vi "Register Process.vi"(0 "Message Handler In":refnum<class "Message Handler.lvclass">, 1 "ProcessRefs":T1, 7 "Process":refnum<class "ICanCommunicate.lvclass">, 11 "Error In":errorcluster) -> (4 "Message Handler Out":refnum<class "Message Handler.lvclass">, 15 "Error Out":errorcluster)   [LabVIEW 2023, in "Message Handler.lvclass"]
uses:
  Message Handler.lvclass
  Interfaces/ICanCommunicate/ICanCommunicate.lvclass
  Interfaces/ICanCommunicate/Process Refs.ctl
  Interfaces/ICanCommunicate/ToProcessQueue.ctl
  Interfaces/ICanCommunicate/Message.ctl
  Interfaces/ICanCommunicate/FromProcessQueue.ctl
  Interfaces/ICanCommunicate/ProcessSyncQueue.ctl
  Private/Ctrls/Registration Data.ctl
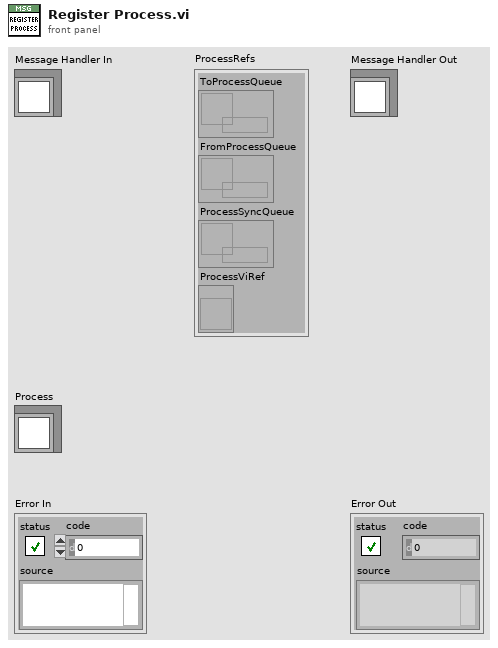
[diagram p1: front panel]
types:
  T1 = typedef "ICanCommunicate.lvclass/Process Refs.ctl" = cluster{"ToProcessQueue":T2, "FromProcessQueue":T3, "ProcessSyncQueue":T4, "ProcessViRef":refnum<vi>}
  T2 = typedef "ICanCommunicate.lvclass/ToProcessQueue.ctl" = refnum<queue>
  T3 = typedef "ICanCommunicate.lvclass/FromProcessQueue.ctl" = refnum<queue>
  T4 = typedef "ICanCommunicate.lvclass/ProcessSyncQueue.ctl" = refnum<queue>
  T5 = typedef "Message Handler.lvclass/Registration Data.ctl" = cluster{"ICanCommunicate":refnum<class "ICanCommunicate.lvclass">, "ProcessRefs":T1}
  T6 = typedef "ICanCommunicate.lvclass/Message.ctl" = cluster{"Sender Name":string, "Recipent Name":string, "Command":string, "Data":variant, "Signature":string}
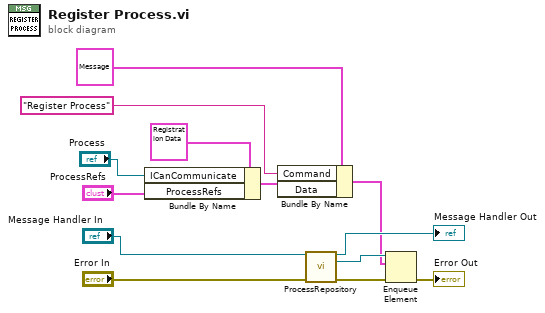
[diagram p0: block diagram]
diagram:
  n1 = Bundle By Name(cluster=T5 {"ICanCommunicate"=refnum, "ProcessRefs"={"ToProcessQueue"=refnum, "FromProcessQueue"=refnum, "ProcessSyncQueue"=refnum, "ProcessViRef"=refnum}} ("Registration Data"), "ICanCommunicate"="Process", "ProcessRefs"="ProcessRefs") -> (w6:T5)
  n2 = Bundle By Name(cluster=T6 {"Sender Name"="", "Recipent Name"="", "Command"="", "Data"=variant, "Signature"=""} ("Message"), "Command"="Register Process", "Data"=w6) -> (w5:T6)
  n3 = call-dynamic "ProcessRepository.vi"("Process In"="Message Handler In", "Error In"="Error In") -> ("Process Out"=→"Message Handler Out":refnum<class "Message Handler.lvclass">, "ToProcessQueue"=w11:T2, "Error Out"=w4:errorcluster)  [unwired: 7 in, 4 out]
  n4 = Enqueue Element(queue=w11, element=w5, error in (no error)=w4) -> (error out=→"Error Out":errorcluster)  [unwired: 1 in, 2 out]
